vi "loop_stop .vi"() -> ()   [LabVIEW 2017]
panel:
  in  "stop 4":bool
  out "Numeric 6":i32
  in  "stop 3":bool
  out "Numeric 5":i32
  out "Numeric 4":i32
  in  "stop 2":bool
  out "Numeric 3":i32
  out "Numeric 2":dbl
  out "Numeric":dbl
  in  "stop":bool
  out "Boolean 8":bool
  out "Boolean 7":bool
  out "Boolean 4":bool
  out "Boolean 3":bool
  out "Boolean 2":bool
  out "1":bool
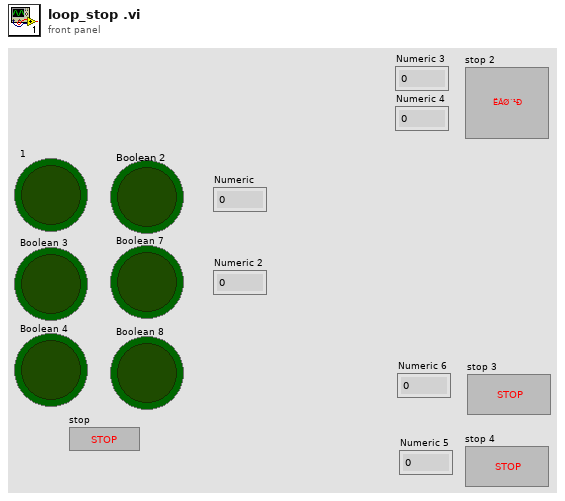
[diagram p1: front panel]
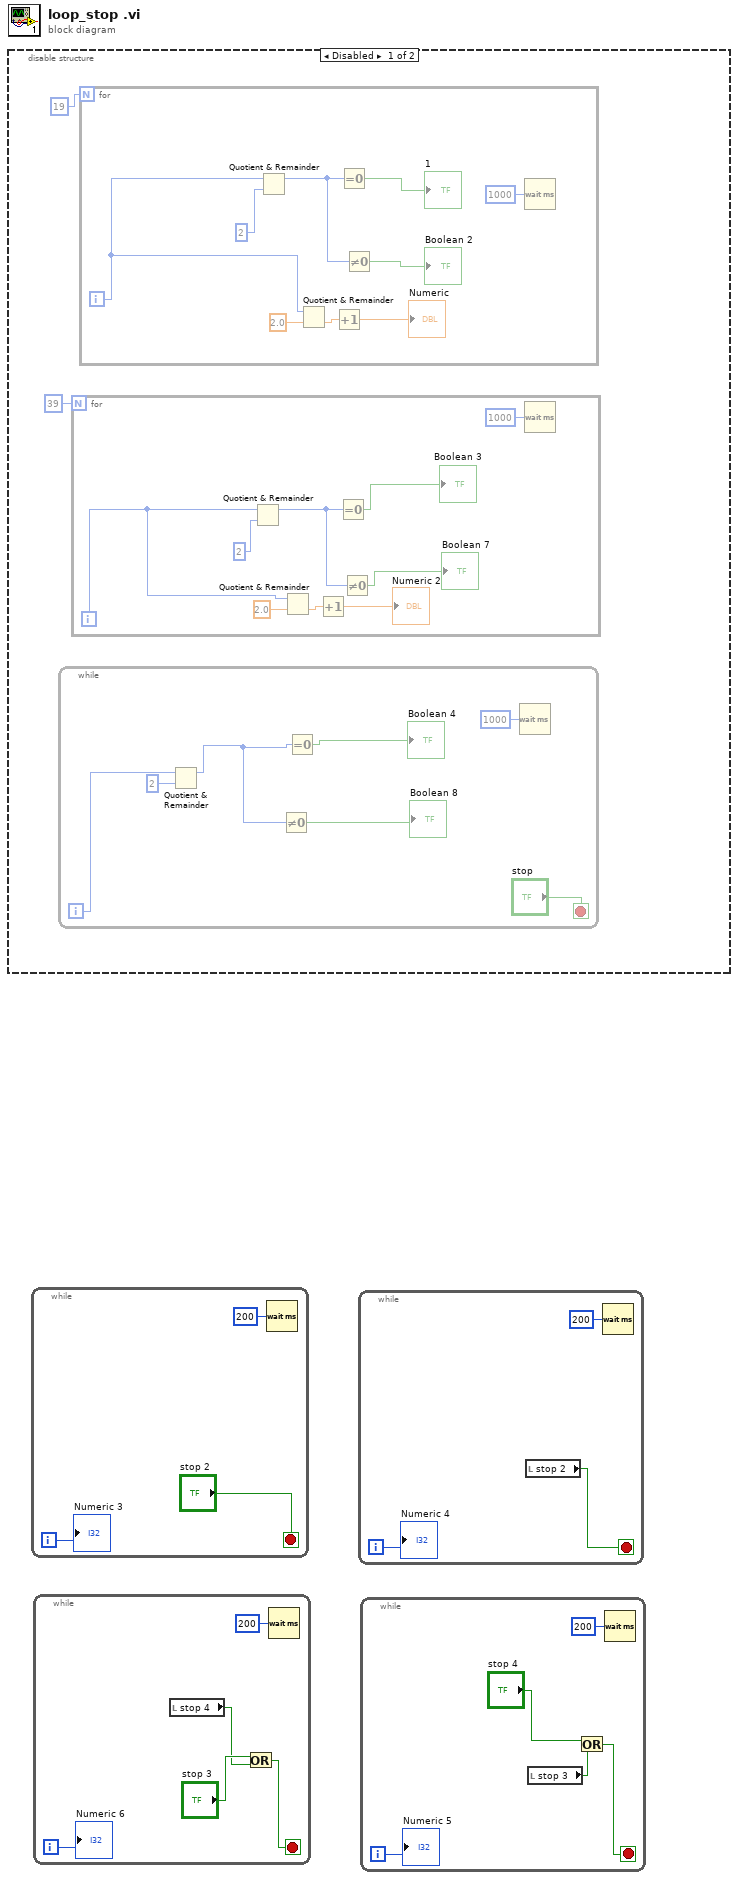
[diagram p0: block diagram]
diagram:
  n1 = disable-structure shown="Disabled" {
    frame Disabled {
      n2 = while {
        i -> [w9]
        stop <- "stop" stop-if-true
        n3 = Quotient & Remainder(x=w9, y=2) -> (x-y*floor(x/y)=w4:i32)  [unwired: 1 out]
        n4 = Not Equal To 0?(x=w4) -> (x != 0?=→"Boolean 8":bool)
        n5 = Equal To 0?(x=w4) -> (x = 0?=→"Boolean 4":bool)
        n6 = Wait (ms)(milliseconds to wait=u32 1000) -> ()  [unwired: 1 out]
      }
      n7 = for {
        N: 39 -> [_]
        i -> [w10]
        n8 = Quotient & Remainder(x=w10, y=2) -> (x-y*floor(x/y)=w18:i32)  [unwired: 1 out]
        n9 = Quotient & Remainder(x=w10, y=2.0) -> (floor(x/y)=w12:dbl)  [unwired: 1 out]
        n10 = Increment(x=w12) -> (x+1=→"Numeric 2":dbl)
        n11 = Equal To 0?(x=w18) -> (x = 0?=→"Boolean 3":bool)
        n12 = Not Equal To 0?(x=w18) -> (x != 0?=→"Boolean 7":bool)
        n13 = Wait (ms)(milliseconds to wait=u32 1000) -> ()  [unwired: 1 out]
      }
      n14 = for {
        N: 19 -> [_]
        i -> [w20]
        n15 = Quotient & Remainder(x=w20, y=2) -> (x-y*floor(x/y)=w24:i32)  [unwired: 1 out]
        n16 = Quotient & Remainder(x=w20, y=2.0) -> (floor(x/y)=w21:dbl)  [unwired: 1 out]
        n17 = Increment(x=w21) -> (x+1=→"Numeric":dbl)
        n18 = Equal To 0?(x=w24) -> (x = 0?=→"1":bool)
        n19 = Not Equal To 0?(x=w24) -> (x != 0?=→"Boolean 2":bool)
        n20 = Wait (ms)(milliseconds to wait=u32 1000) -> ()  [unwired: 1 out]
      }
    }
    frame Enabled {
    }
  }
  n21 = while {
    i -> [w30]
    stop <- "stop 2" stop-if-true
    n22 = Wait (ms)(milliseconds to wait=u32 200) -> ()  [unwired: 1 out]
    "Numeric 3" <- w30
  }
  n23 = while {
    i -> [w35]
    stop <- w33 stop-if-true
    n24 = local read "stop 4"() -> (w31:bool)
    n25 = Or(x="stop 3", y=w31) -> (x .or. y?=w33:bool)
    n26 = Wait (ms)(milliseconds to wait=u32 200) -> ()  [unwired: 1 out]
    "Numeric 6" <- w35
  }
  n27 = while {
    i -> [w38]
    stop <- w36 stop-if-true
    n28 = local read "stop 2"() -> (w36:bool)
    n29 = Wait (ms)(milliseconds to wait=u32 200) -> ()  [unwired: 1 out]
    "Numeric 4" <- w38
  }
  n30 = while {
    i -> [w43]
    stop <- w39 stop-if-true
    n31 = local read "stop 3"() -> (w40:bool)
    n32 = Or(x="stop 4", y=w40) -> (x .or. y?=w39:bool)
    n33 = Wait (ms)(milliseconds to wait=u32 200) -> ()  [unwired: 1 out]
    "Numeric 5" <- w43
  }
